vi "Create Map Entries.vi"(8 "error in (no error)":errorcluster, 11 "LV-Protoc in":refnum<class "LV-Protoc.lvclass">) -> (0 "error out":errorcluster, 3 "LV-Protoc out":refnum<class "LV-Protoc.lvclass">)   [LabVIEW 2020, in "LV-Protoc.lvlib" / "LV-Protoc.lvclass"]
doc: "Creates message definitions to replace map definitions with. In protobuf, maps are just repeated message entries where the nested messages contain key and value fields."
uses:
  LV-Protoc.lvclass
  LV-Protoc.lvclass/LV-Protoc.ctl
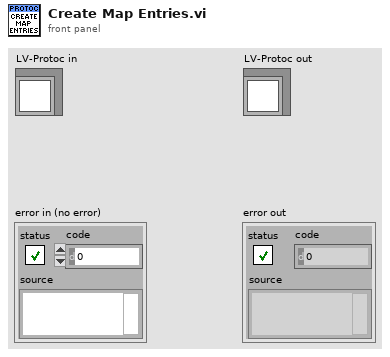
[diagram p1: front panel]
types:
  T1 = typedef "LV-Protoc.lvlib/Map Definition.ctl" = cluster{"Message":string, "Definition":T2}
  T2 = typedef "LV-Proto.lvlib/Field.ctl" = cluster{"Name":string, "Number":u32, "Optional":bool, "Repeated":bool, "Type":T3, "Key Type":T3, "Value Type":T3}
  T3 = typedef "LV-Proto.lvlib/Type.ctl" = cluster{"Type":T4, "Subtype":string}
  T4 = typedef "LV-Proto.lvlib/Proto Type.ctl" = enum16{"UNKNOWN", "double", "float", "int32", "int64", "uint32", "uint64", "sint32", "sint64", "fixed32", "fixed64", "sfixed32", "sfixed64", "bool", "string", "bytes", "enum", "map", "message"}
  T5 = typedef "LV-Proto.lvlib/Message.ctl" = cluster{"Name":string, "Fields":T2[], "Reserved Numbers":u32[], "Reserved Names":string[]}
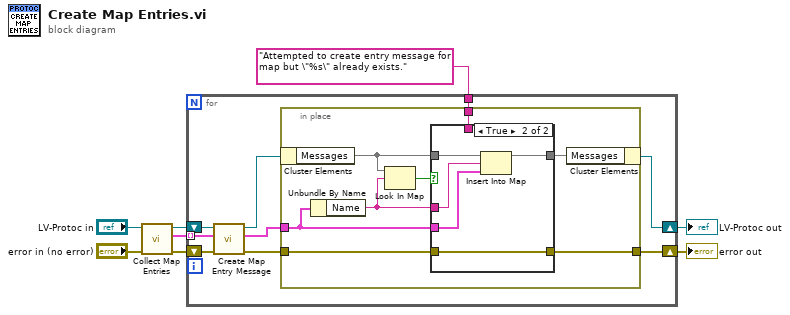
[diagram p0: block diagram]
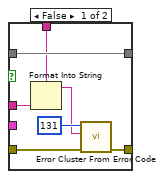
[diagram p2: hidden frame]
diagram:
  n1 = call "Collect Map Entries.vi"("error in (no error)"="error in (no error)", "LV-Protoc in"="LV-Protoc in") -> ("error out"=w5:errorcluster, "Map Fields"=w4:T1[], "LV-Protoc out"=w6:refnum<class "LV-Protoc.lvclass">)  [unwired: 7 in]
  n2 = for {
    shift-right: [w9] -> w3
    shift-left: w6 -> [w17]
    shift-right: [w10] -> w2
    shift-left: w5 -> [w16]
    tunnel: w4 -> [w15] mode=indexing
    tunnel: "Attempted to create entry message for map but \"%s\" already exists." -> [w11]
    n3 = call "Create Map Entry Message.vi"("error in (no error)"=w16, "Map Definition"=w15, "LV-Protoc in"=w17) -> ("error out"=w12:errorcluster, "Message"=w13:T5, "LV-Protoc out"=w14:refnum<class "LV-Protoc.lvclass">)  [unwired: 6 in]
    n4 = in-place {
      in-place-border: w13 -> [w22]
      in-place-border: w12 -> [w20]
      in-place-border: w11 -> [w19]
      in-place-border: [w18] -> w10
      n5 = in-place-cluster #1(w14) -> ("Messages"=w24:map{string, T5})
      n6 = Unbundle By Name(w22) -> ("Name"=w23:string)
      n7 = Look In Map(map=w24, key=w23) -> (key not found?=w25:bool)  [unwired: 1 in, 1 out]
      n8 = case shown="True" w25 {
        tunnel: w24 -> [w32 w37]
        tunnel: w23 -> [w28 w35]
        tunnel: w22 -> [_ w34]
        tunnel: [w32 w36] -> w21
        tunnel: w20 -> [w31 w33]
        tunnel: w19 -> [w29 _]
        tunnel: [w26 w33] -> w18
        frame False {
          n9 = Format Into String(format string=w29, w28) -> (resulting string=w27:string)  [unwired: 2 in, 1 out]
          n10 = call <vilib>:"Error Cluster From Error Code.vi"("error in (no error)"=w31, "error message (\"\")"=w27, "error code (0)"=131) -> ("error out"=w26:errorcluster)  [unwired: 6 in]
        }
        frame True {
          n11 = Insert Into Map(map in=w37, key=w35, value=w34) -> (map out=w36:map{string, T5})  [unwired: 2 out]
        }
      }
      n12 = in-place-cluster #1("Messages"=w21) -> (w9:refnum<class "LV-Protoc.lvclass">)
    }
  }
  "error out" <- w2
  "LV-Protoc out" <- w3
